vi "DEVICE_ID_LENGTH.vi"() -> (3 "DEVICE_ID_LENGTH":i32=256)   [LabVIEW 2020, in "G-Audio.lvlib"]
uses:
  G-Audio.lvlib
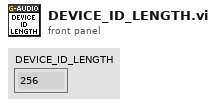
[diagram p1: front panel]
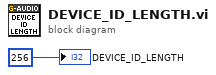
[diagram p0: block diagram]
diagram:
  "DEVICE_ID_LENGTH" <- 256
